vi "Begin.vi"(8 "error in":errorcluster) -> (0 "error out":errorcluster)   [LabVIEW 2018]
doc: "Called before other user functions, this VI is expected to open initial I/O refnums, load in file data, and do all program initialization. Notice that the <B>error out</B> terminal is simply used for data flow. Wiring it to other structures or subVIs ensures that this VI runs first."
uses:
  LeftMotors.ctl
  RightMotors.ctl
  <vilib>/Utility/file.llb/Read Delimited Spreadsheet (DBL).vi
  Robot Global Data.vi
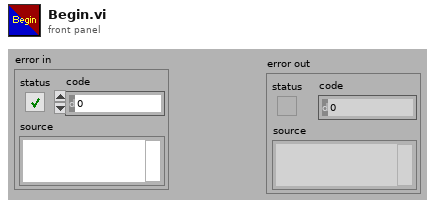
[diagram p1: front panel]
types:
  T1 = typedef "RightMotors.ctl" = enum16{"RightMotor1", "RightMotor2", "RightMotor3"}
  T2 = typedef "LeftMotors.ctl" = enum16{"LeftMotor1", "LeftMotor2", "LeftMotor3"}
  T3 = typedef "WPI_MotorControlDeviceRef.ctl" = cluster{"DeviceStatus":errorcluster, "Type":T4, "PWM":cluster{"PWM Channel":T5, "DeadBand":T6}, "CAN":cluster{"Device Number":u8, "SetOutput VI Ref":variant, "GetOutput VI Ref":variant, "Enable VI Ref":variant, "Disable VI Ref":variant, "Data":variant}, "Invert":bool, "DIO PWM":cluster{"PWM \"Enable\" Channel":T5, "DIOChannel":T7, "PWM Rate":dbl}}
  T4 = typedef "WPI_MotorControlType.ctl" = enum16{"PWM", "CAN", "DIO PWM"}
  T5 = typedef "FPGA_DIOPWMChannel.ctl" = enum8{"PWM 0", "PWM 1", "PWM 2", "PWM 3", "PWM 4", "PWM 5", "PWM 6", "PWM 7", "PWM 8", "PWM 9", "PWM MXP 0", "PWM MXP 1", "PWM MXP 2", "PWM MXP 3", "PWM MXP 4", "PWM MXP 5", "PWM MXP 6", "PWM MXP 7", "PWM MXP 8", "PWM MXP 9", "Invalid"}
  T6 = typedef "WPI_PWMDeadband.ctl" = cluster{"Name":string, "maxPositivePwm":i32, "minPositivePwm":i32, "centerPwm":i32, "maxNegativePwm":i32, "minNegativePwm":i32, "angularRange":u16}
  T7 = typedef "FPGA_DIOChannel.ctl" = enum8{"DIO 0", "DIO 1", "DIO 2", "DIO 3", "DIO 4", "DIO 5", "DIO 6", "DIO 7", "DIO 8", "DIO 9", "DIO MXP 0", "DIO MXP 1", "DIO MXP 2", "DIO MXP 3", "DIO MXP 4", "DIO MXP 5", "DIO MXP 6", "DIO MXP 7", "DIO MXP 8", "DIO MXP 9", "DIO MXP 10", "DIO MXP 11", "DIO MXP 12", "DIO MXP 13", "DIO MXP 14", "DIO MXP 15", "SPI Port CS1", "SPI Port CS2", "SPI Port CS3", "SPI Port MISO", "SPI Port MOSI", "Invalid"}
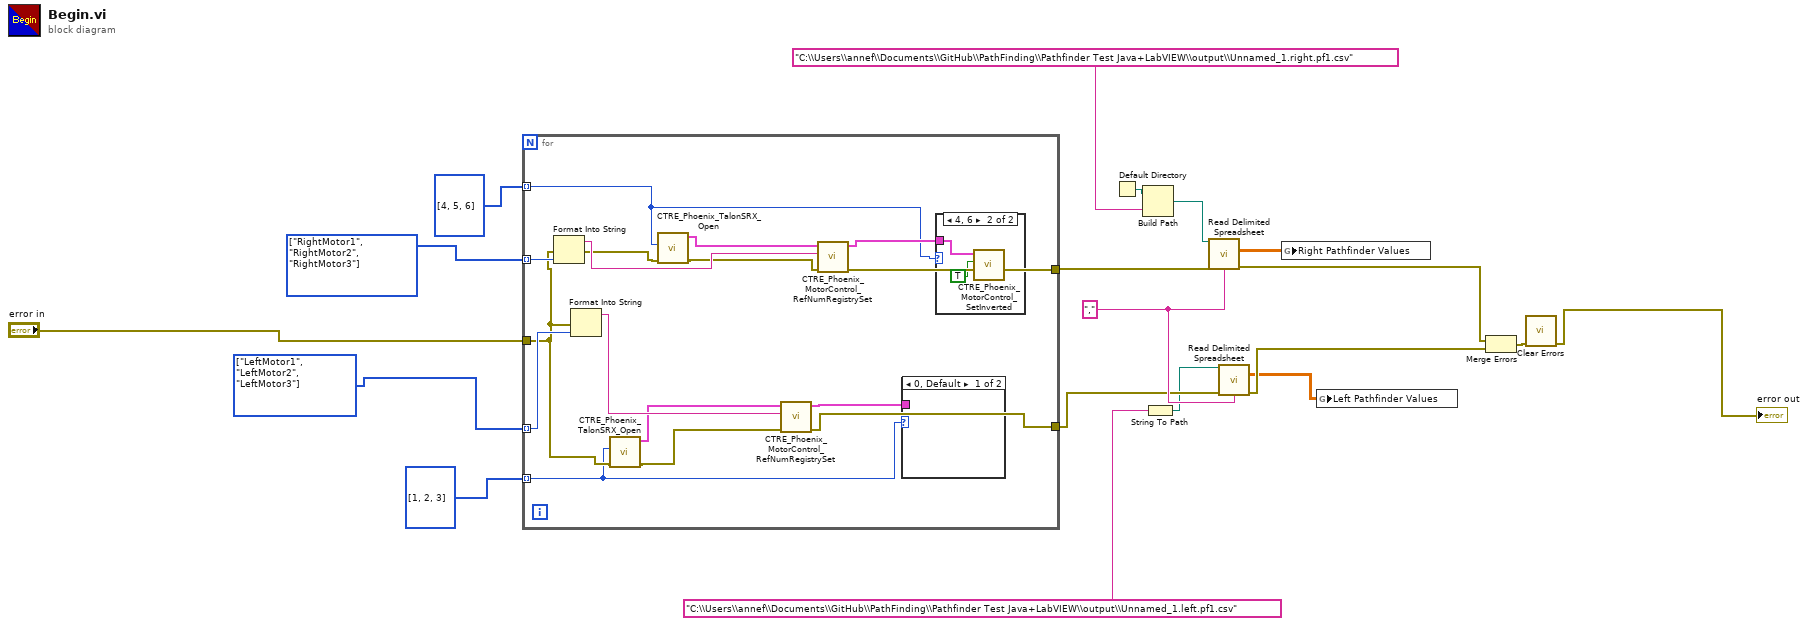
[diagram p0: block diagram]
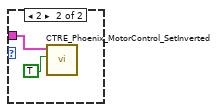
[diagram p2: hidden frame]
diagram:
  w11 = "," ("delimiter (\\t)")
  w15 = T1[] [enum."RightMotor1", enum."RightMotor2", enum."RightMotor3"] items=["RightMotor1", "RightMotor2", "RightMotor3"]
  w14 = T2[] [enum."LeftMotor1", enum."LeftMotor2", enum."LeftMotor3"] items=["LeftMotor1", "LeftMotor2", "LeftMotor3"]
  n1 = for {
    tunnel: w14 -> [w35] mode=indexing
    tunnel: "error in" -> [w27]
    tunnel: [w30] -> w10
    tunnel: w15 -> [w33] mode=indexing
    tunnel: [w31] -> w12
    tunnel: u8[] [1, 2, 3] ("Device Number") -> [w20] mode=indexing
    tunnel: u8[] [4, 5, 6] ("Device Number") -> [w22] mode=indexing
    n2 = Format Into String(error in=w27, w33) -> (resulting string=w32:string, error out=w24:errorcluster)  [unwired: 2 in]
    n3 = Format Into String(error in=w27, w35) -> (resulting string=w34:string)  [unwired: 2 in, 1 out]
    n4 = call <vilib>:"CTRE_Phoenix_TalonSRX_Open.vi"("error in"=w27, "Device Number"=w20) -> ("error out"=w28:errorcluster, "CAN Talon SRX Ref"=w29:T3)  [unwired: 8 in]
    n5 = call <vilib>:"CTRE_Phoenix_TalonSRX_Open.vi"("error in"=w24, "Device Number"=w22) -> ("error out"=w25:errorcluster, "CAN Talon SRX Ref"=w26:T3)  [unwired: 8 in]
    n6 = call <vilib>:"CTRE_Phoenix_MotorControl_RefNumRegistrySet.vi"("error in (no error)"=w28, "refnum name"=w34, "PhoenixMotorControlDevRef"=w29) -> ("error out"=w30:errorcluster, "PhoenixMotorControlDevRef"=w21:T3)  [unwired: 7 in]
    n7 = call <vilib>:"CTRE_Phoenix_MotorControl_RefNumRegistrySet.vi"("error in (no error)"=w25, "refnum name"=w32, "PhoenixMotorControlDevRef"=w26) -> ("error out"=w31:errorcluster, "PhoenixMotorControlDevRef"=w23:T3)  [unwired: 7 in]
    n8 = case shown="0, Default" w20 {
      tunnel: w21 -> [_ w37]
      frame 0, Default {
      }
      frame 2 {
        n9 = call <vilib>:"CTRE_Phoenix_MotorControl_SetInverted.vi"("Invert?"=TRUE, "PhoenixMotorControlDevRef"=w37) -> ()  [unwired: 8 in, 2 out]
      }
    }
    n10 = case shown="4, 6" w22 {
      tunnel: w23 -> [_ w39]
      frame 0, Default {
      }
      frame 4, 6 {
        n11 = call <vilib>:"CTRE_Phoenix_MotorControl_SetInverted.vi"("Invert?"=TRUE, "PhoenixMotorControlDevRef"=w39) -> ()  [unwired: 8 in, 2 out]
      }
    }
  }
  n12 = Default Directory() -> (w3:path)
  n13 = Build Path(base path=w3, name or relative path="C:\\Users\\annef\\Documents\\GitHub\\PathFinding\\Pathfinder Test Java+LabVIEW\\output\\Unnamed_1.right.pf1.csv" ("string")) -> (appended path=w1:path)
  n14 = String To Path(string="C:\\Users\\annef\\Documents\\GitHub\\PathFinding\\Pathfinder Test Java+LabVIEW\\output\\Unnamed_1.left.pf1.csv") -> (path=w4:path)
  n15 = call-poly <vilib>:"Read Delimited Spreadsheet.vi"("file path (dialog if empty)"=w1, "error in (no error)"=w12, "delimiter (\\t)"=w11) -> ("all rows"=w7:dbl[][], "error out"=w8:errorcluster)  [unwired: 7 in, 4 out]
  n16 = call-poly <vilib>:"Read Delimited Spreadsheet.vi"("file path (dialog if empty)"=w4, "error in (no error)"=w10, "delimiter (\\t)"=w11) -> ("all rows"=w6:dbl[][], "error out"=w9:errorcluster)  [unwired: 7 in, 4 out]
  n17 = global write "Robot Global Data.vi" "Right Pathfinder Values"(w7) -> ()
  n18 = global write "Robot Global Data.vi" "Left Pathfinder Values"(w6) -> ()
  n19 = Merge Errors(w8, w9) -> (w17:errorcluster)
  n20 = call <vilib>:"Clear Errors.vi"("error in (no error)"=w17) -> ("error out"=→"error out":errorcluster)  [unwired: 5 in, 1 out]
